vi "Windmill_interlock.vi"(8 "error in (no error)":errorcluster, 11 "WindmillDevice in":refnum<class "WindmillDevice.lvclass">) -> (0 "error out":errorcluster, 3 "WindmillDevice out":refnum<class "WindmillDevice.lvclass">)   [LabVIEW 2020, in "WindmillDevice.lvclass"]
uses:
  WindmillDevice.lvclass
  WindmillDevice.lvclass/WindmillDevice.ctl
panel:
  out "MonitorCheck":enum16{"off", "on"}(ring)
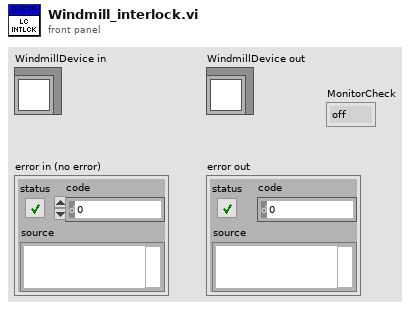
[diagram p1: front panel]
types:
  T1 = typedef "SubscriberCluster_TypDEf.ctl" = cluster{"tcp data event":T2, "Event Registration Refnum":refnum<event-registration>, "data queue":refnum<queue>, "Devices":string[], "Alias":string[], "Variable header":string[], "Devices ALL":string[]}
  T2 = typedef "tcp_new_data_event.ctl" = refnum<user-event>
  T3 = cluster{"MonMaxCounts":dbl, "MonMeanCountsRaw":dbl}
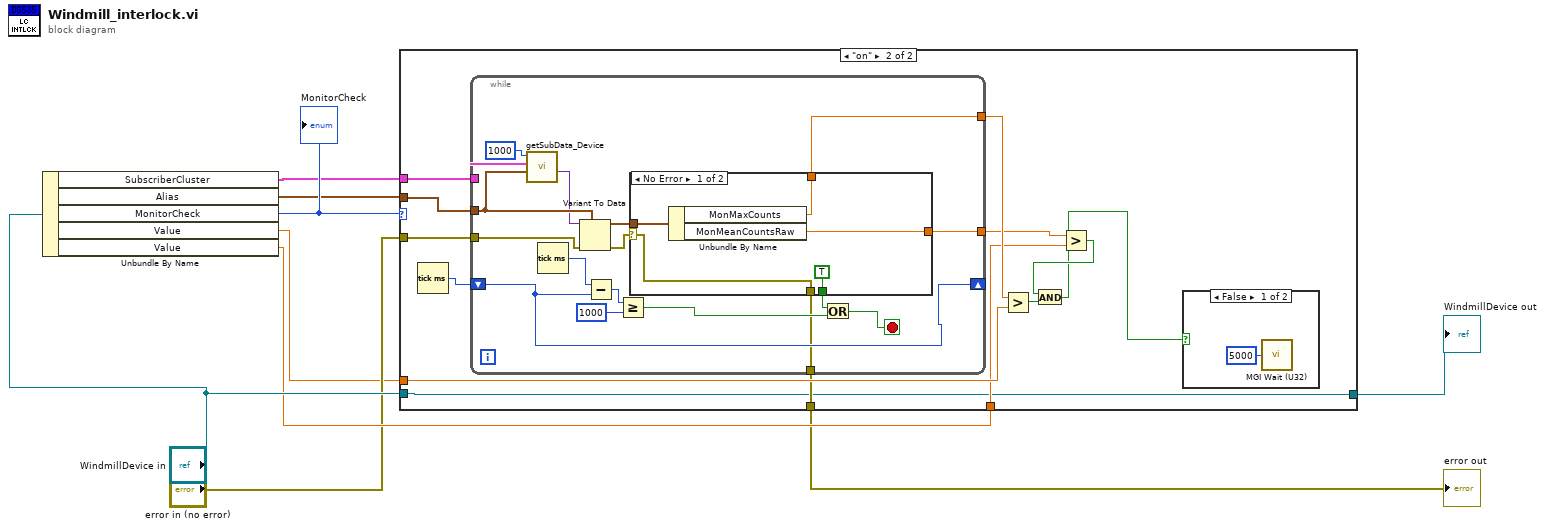
[diagram p0: block diagram]
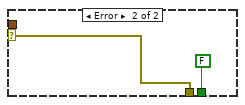
[diagram p4: hidden frame]
diagram:
  n1 = Unbundle By Name("WindmillDevice in") -> ("SubscriberCluster"=w2:T1, "Alias"=w1:T3, "MonitorCheck"=w6:enum16{"off", "on"}, "Value"=w3:dbl, "Value"=w7:dbl)
  "MonitorCheck" <- w6
  n2 = case shown="\"on\"" w6 {
    tunnel: w1 -> [_ w24]
    tunnel: w2 -> [_ w23]
    tunnel: w3 -> [_ w20]
    tunnel: "error in (no error)" -> [w11 w19]
    tunnel: [w11 w18] -> w5
    tunnel: w7 -> [_ w13]
    tunnel: "WindmillDevice in" -> [w10 w12]
    tunnel: [w10 w12] -> w9
    frame "off", Default {
    }
    frame "on" {
      n3 = Tick Count (ms)() -> (millisecond timer value=w22:u32)
      n4 = while {
        tunnel: w24 -> [w42]
        tunnel: w23 -> [w41]
        shift-right: [w32] -> _
        shift-left: w22 -> [w32]
        tunnel: [w29] -> w21
        tunnel: w19 -> [w28]
        tunnel: [w27] -> w18
        tunnel: [w26] -> w17
        stop <- w33 stop-if-true
        n5 = call "getSubData_Device.vi"("variant in"=w42, "SubscriberCluster"=w41, "timeout"=1000) -> ("variant out"=w39:variant)  [unwired: 6 in, 2 out]
        n6 = Tick Count (ms)() -> (millisecond timer value=w37:u32)
        n7 = Variant To Data(error in=w28, type=w42, Variant=w39) -> (data=w40:T3, error out=w31:errorcluster)
        n8 = Subtract(x=w37, y=w32) -> (x-y=w36:u32)
        n9 = Greater Or Equal?(x=w36, y=u32 1000) -> (x >= y?=w34:bool)
        n10 = case shown="No Error" w31 {
          selector: w31 -> [w44 w48]
          tunnel: w40 -> [w47 _]
          tunnel: [TRUE FALSE] -> w30
          tunnel: [w45 _] -> w29
          tunnel: [w44 w48] -> w27
          tunnel: [w43 _] -> w26
          frame No Error {
            n11 = Unbundle By Name(w47) -> ("MonMaxCounts"=w45:dbl, "MonMeanCountsRaw"=w43:dbl)
          }
          frame Error {
          }
        }
        n12 = Or(x=w30, y=w34) -> (x .or. y?=w33:bool)
      }
      n13 = Greater?(x=w21, y=w20) -> (0:w16:bool)
      n14 = Greater?(x=w17, y=w13) -> (0:w15:bool)
      n15 = And(x=w15, y=w16) -> (x .and. y?=w14:bool)
      n16 = case shown="False" w14 {
        frame False {
          n17 = call "MGI Wait (U32).vi"("ms"=u32 5000 ("WaitBeforeScanStep_ms")) -> ()  [unwired: 6 in, 1 out]
        }
        frame True {
        }
      }
    }
  }
  "WindmillDevice out" <- w9
  "error out" <- w5
